vi "Remove VI.vi"(8 "error in (no error)":errorcluster, 10 "VI Name":string, 11 "ProjectData in":refnum<class "Project Data.lvclass">) -> (0 "error out":errorcluster, 1 "Removed VI":refnum<class "VI Data.lvclass">, 2 "found":bool, 3 "ProjectData out":refnum<class "Project Data.lvclass">)   [LabVIEW 2013, in "SET Project Data.lvlib" / "Project Data.lvclass"]
uses:
  Project Data.lvclass
  VI Class/VI Data.lvclass
  Project Data.lvclass/Project Data.ctl
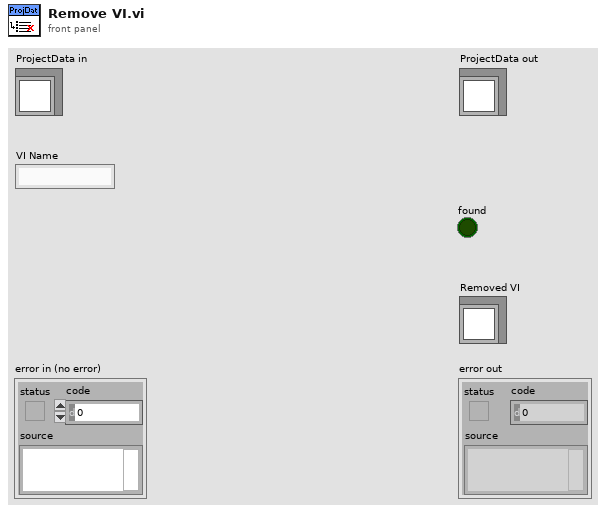
[diagram p1: front panel]
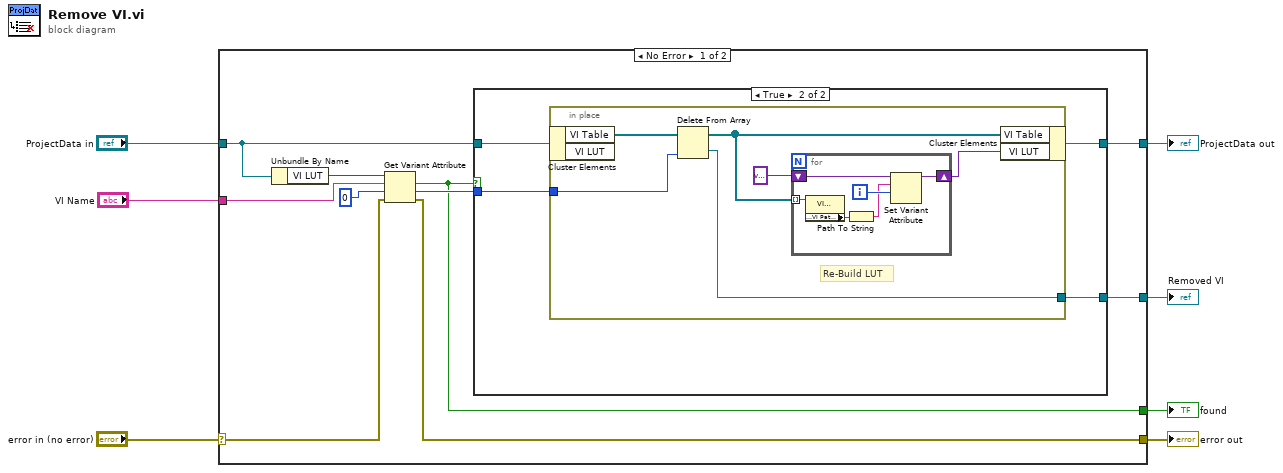
[diagram p0: block diagram]
diagram:
  n1 = case shown="No Error" "error in (no error)" {
    selector: "error in (no error)" -> [w14 w36]
    tunnel: [w13 w36] -> w6
    tunnel: [w10 w35] -> w4
    tunnel: "ProjectData in" -> [w11 w35]
    tunnel: "VI Name" -> [w16 _]
    tunnel: [w9 _] -> w2
    tunnel: [w8 _] -> w1
    frame No Error {
      n2 = Unbundle By Name(w11) -> ("VI LUT"=w17:variant)
      n3 = Get Variant Attribute(Variant=w17, name=w16, default value (empty Variant)=0, error in=w14) -> (found=w9:bool, value=w12:i32, error out=w13:errorcluster)  [unwired: 1 out]
      n4 = case shown="True" w9 {
        tunnel: w12 -> [_ w22]
        tunnel: w11 -> [w18 w21]
        tunnel: [w18 w20] -> w10
        tunnel: [_ w19] -> w8
        frame False {
        }
        frame True {
          n5 = in-place {
            in-place-border: w22 -> [w27]
            in-place-border: [w26] -> w19
            # "Re-Build LUT"
            n6 = in-place-cluster #1(w21) -> ("VI Table"=w28:refnum<class "VI Data.lvclass">[])  [unwired: 1 out]
            n7 = Delete From Array(array=w28, index=w27) -> (deleted portion=w26:refnum<class "VI Data.lvclass">, array with subset deleted=w25:refnum<class "VI Data.lvclass">[])  [unwired: 1 in]
            n8 = for {
              tunnel: w25 -> [w32] mode=indexing
              shift-right: [w33] -> w23
              shift-left: variant ("type") -> [w34]
              i -> [w31]
              n9 = property class="VI Data.lvclass"(reference=w32) -> ("Properties:VI Path (Relative)"=w30:path)  [unwired: 1 in, 2 out]
              n10 = Path To String(path=w30) -> (string=w29:string)
              n11 = Set Variant Attribute(Variant=w34, name=w29, value=w31) -> (Variant out=w33:variant)  [unwired: 1 in, 2 out]
            }
            n12 = in-place-cluster #1("VI Table"=w25, "VI LUT"=w23) -> (w20:refnum<class "Project Data.lvclass">)
          }
        }
      }
    }
    frame Error {
    }
  }
  "error out" <- w6
  "ProjectData out" <- w4
  "found" <- w2
  "Removed VI" <- w1
